vi "test filter by name.vi"() -> ()   [LabVIEW 2013, in "TBM Tests.lvlib"]
uses:
  TBM Tests.lvlib
  <vilib>/NI/Tag Bus/tag/tag descriptor.lvclass/tag descriptor.ctl
  channel/TBM channel.lvclass/TBM channel.ctl
  <vilib>/NI/Tag Bus/tag/read tag name.vi
  <vilib>/NI/Tag Bus/tag/read data type.vi
  channel/Read channel classification.vi
  channel/TBM channel.lvclass
panel:
  out "filter ok":bool
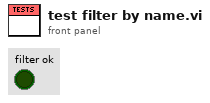
[diagram p1: front panel]
types:
  T1 = typedef "TBM channel.lvclass/channel classification.ctl" = enum16{"input data", "output data", "processing parameter", "processing result"}
  T2 = typedef "tag bus.lvlib/tag descriptor.lvclass/Data Type.ctl" = enum16{"Double", "Single", "I64", "I32", "I16", "I8", "U64", "U32", "U16", "U8", "Boolean", "String", "Array of Double", "Array of Single", "Array of I64", "Array of I32", "Array of I16", "Array of I8", "Array of U64", "Array of U32", "Array of U16", "Array of U8", "Array of Boolean", "Array of String"}
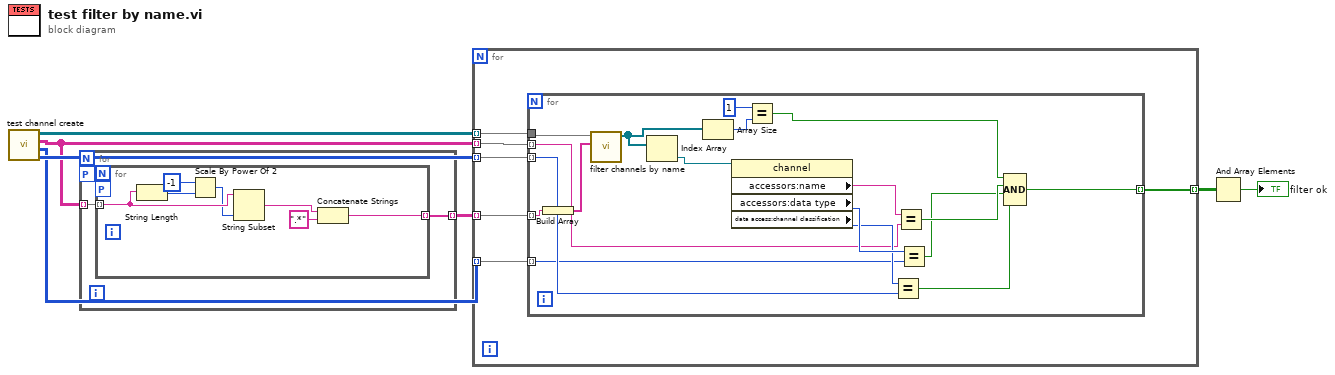
[diagram p0: block diagram]
diagram:
  n1 = call "test channel create.vi"() -> ("dirs"=w4:T1[][], "types"=w3:T2[][], "names"=w2:string[][], "chans"=w7:refnum<class "TBM channel.lvclass">[][])  [unwired: 8 in]
  n2 = for {
    tunnel: w2 -> [w9] mode=indexing
    tunnel: [w8] -> w1 mode=indexing
    workers-P: _ -> [_]
    n3 = for {
      tunnel: w9 -> [w14] mode=indexing
      tunnel: [w10] -> w8 mode=indexing
      workers-P: _ -> [_]
      n4 = String Length(string=w14) -> (length=w16:i32)
      n5 = Scale By Power Of 2(n=i16 -1, x=w16) -> (x*2^n=w13:i32)
      n6 = String Subset(string=w14, length (rest)=w13) -> (substring=w12:string)  [unwired: 1 in]
      n7 = Concatenate Strings(w12, ".*" ("string")) -> (w10:string)
    }
  }
  n8 = for {
    tunnel: w7 -> [w22] mode=indexing
    tunnel: w2 -> [w21] mode=indexing
    tunnel: [w20] -> w6 mode=indexing
    tunnel: w4 -> [w19] mode=indexing
    tunnel: w3 -> [w18] mode=indexing
    tunnel: w1 -> [w17] mode=indexing
    n9 = for {
      tunnel: w22 -> [w28]
      tunnel: w21 -> [w31] mode=indexing
      tunnel: [w37] -> w20 mode=indexing
      tunnel: w19 -> [w33] mode=indexing
      tunnel: w18 -> [w32] mode=indexing
      tunnel: w17 -> [w30] mode=indexing
      n10 = Build Array(w30) -> (w29:string[])
      n11 = call "filter channels by name.vi"("allowed name patterns"=w29, "channels in"=w28) -> ("channels out"=w26:refnum<class "TBM channel.lvclass">[])  [unwired: 9 in]
      n12 = Index Array(array=w26) -> (element=w27:refnum<class "TBM channel.lvclass">)  [unwired: 1 in]
      n13 = Array Size(array=w26) -> (size(s)=w25:i32)
      n14 = property class="channel"(reference=w27) -> ("accessors:name"=w36:string, "accessors:data type"=w35:T2, "data access:channel classification"=w34:T1)  [unwired: 1 in, 2 out]
      n15 = Equal?(x=1, y=w25) -> (x = y?=w23:bool)
      n16 = Equal?(x=w34, y=w33) -> (x = y?=w38:bool)
      n17 = Equal?(x=w36, y=w31) -> (x = y?=w40:bool)
      n18 = Equal?(x=w35, y=w32) -> (x = y?=w39:bool)
      n19 = Compound Arithmetic op=AND(w23, w40, w39, w38) -> (w37:bool)
    }
  }
  n20 = And Array Elements(Boolean array=w6) -> (logical AND=→"filter ok":bool)
